vi "RoboRealmCommunications.vi"() -> ()   [LabVIEW 2013]
panel:
  out "String":string
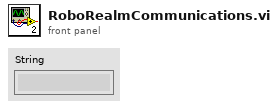
[diagram p1: front panel]
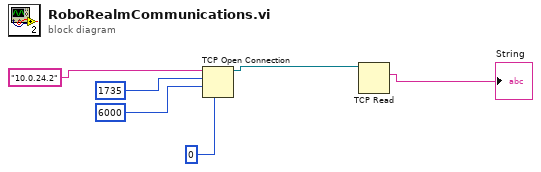
[diagram p0: block diagram]
diagram:
  n1 = TCP Open Connection(address="10.0.24.2", remote port or service name=1735, timeout ms (60000)=6000, local port=0) -> (connection ID=w6:refnum<k5>)  [unwired: 1 in, 1 out]
  n2 = TCP Read(connection ID=w6) -> (data out=→"String":string)  [unwired: 4 in, 2 out]
